vi "test_VISA Close.vi"(8 "error in (no error)":errorcluster, 11 "TestCase in":refnum<class "Instrument Addon Serial Protocols Unit Tests.lvclass">) -> (0 "error out":errorcluster, 3 "TestCase out":refnum<class "Instrument Addon Serial Protocols Unit Tests.lvclass">)   [LabVIEW 2023, in "Instrument Addon Serial Protocols Unit Tests.lvclass"]
uses:
  Instrument Addon Serial Protocols Unit Tests.lvclass
  <vilib>/addons/_JKI Toolkits/VI Tester/TestCase.llb/TestCase.lvclass
  VISA/VISA.lvclass
  Listener/Listener.lvclass
  Listener/ListenerClassControls/Operation.ctl
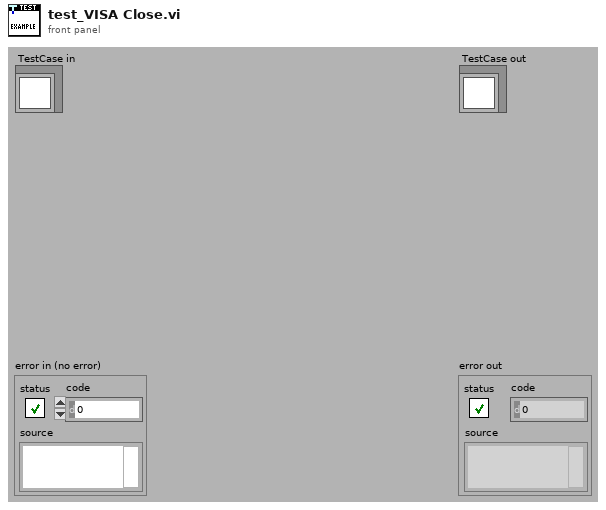
[diagram p1: front panel]
types:
  T1 = typedef "Listener.lvclass/Operation.ctl" = enum16{"Read", "Write"}
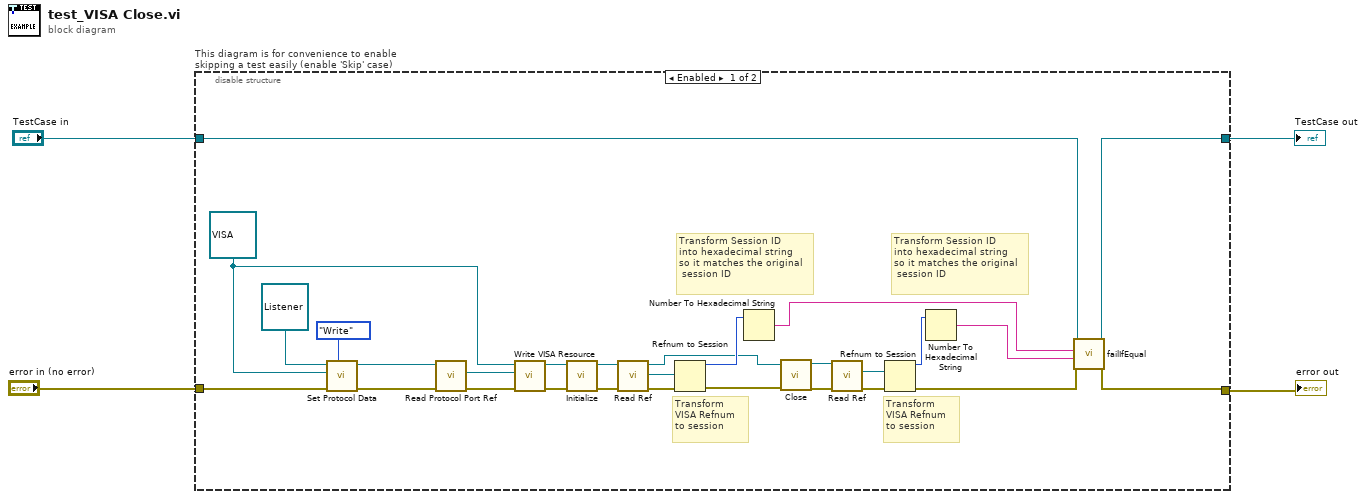
[diagram p0: block diagram]
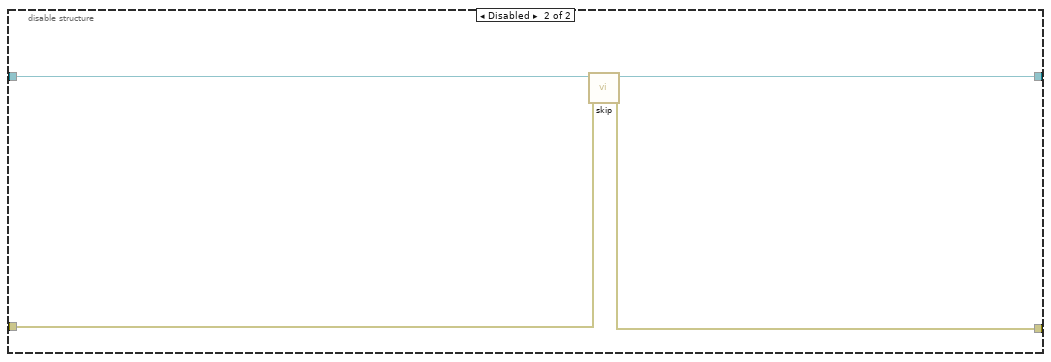
[diagram p2: hidden frame]
diagram:
  n1 = disable-structure "This diagram is for convenience to enable skipping a test easily (enable 'Skip' case)" shown="Enabled" {
    disable-tunnel: "TestCase in" -> [w32 w36]
    disable-tunnel: [w31 w34] -> w1
    disable-tunnel: [w30 w35] -> w3
    disable-tunnel: "error in (no error)" -> [w27 w33]
    frame Enabled {
      w26 = refnum<class "VISA.lvclass"> refnum ("Protocols.lvlib:VISA.lvclass")
      # "Transform Session ID \ninto hexadecimal string\nso it matches the original\n session ID"
      # "Transform \nVISA Refnum \nto session"
      # "Transform Session ID \ninto hexadecimal string\nso it matches the original\n session ID"
      # "Transform \nVISA Refnum \nto session"
      n2 = call "Set Protocol Data.vi"("Operation"=Operation."Write", "error in (no error)"=w27, "Protocols.lvlib:Protocol Parent.lvclass"=w26, "Listener In.lvclass"=refnum<class "Listener.lvclass"> refnum ("Listener.lvclass")) -> ("error out"=w7:errorcluster, "Listener Out.lvclass"=w8:refnum<class "Listener.lvclass">)  [unwired: 6 in]
      n3 = call "Read Protocol Port Ref.vi"("error in (no error)"=w7, "Listener in"=w8) -> ("error out"=w6:errorcluster, "Protocol Port Ref"=w5:refnum<visa-resource-name>)  [unwired: 7 in, 1 out]
      n4 = call "Write VISA Resource.vi"("error in (no error)"=w6, "VISA Resource"=w5, "VISA in"=w26) -> ("error out"=w25:errorcluster, "VISA out"=w24:refnum<class "VISA.lvclass">)  [unwired: 7 in]
      n5 = call-dynamic "Initialize.vi"("error in (no error)"=w25, "VISA in"=w24) -> ("error out"=w23:errorcluster, "VISA out"=w22:refnum<class "VISA.lvclass">)  [unwired: 8 in]
      n6 = call "Read Ref.vi"("error in (no error)"=w23, "VISA in"=w22) -> ("error out"=w18:errorcluster, "Ref"=w21:refnum<visa-resource-name>, "VISA out"=w9:refnum<class "VISA.lvclass">)  [unwired: 7 in]
      n7 = Refnum to Session(4:w18, 7:w21) -> (0:w17:errorcluster, 3:w20:u64)
      n8 = Number To Hexadecimal String(2:w20) -> (0:w10:string)  [unwired: 1 in]
      n9 = call-dynamic "Close.vi"("error in (no error)"=w17, "VISA in"=w9) -> ("error out"=w16:errorcluster, "VISA out"=w19:refnum<class "VISA.lvclass">)  [unwired: 8 in]
      n10 = call "Read Ref.vi"("error in (no error)"=w16, "VISA in"=w19) -> ("error out"=w15:errorcluster, "Ref"=w13:refnum<visa-resource-name>)  [unwired: 7 in, 1 out]
      n11 = Refnum to Session(4:w15, 7:w13) -> (0:w14:errorcluster, 3:w12:u64)
      n12 = Number To Hexadecimal String(2:w12) -> (0:w11:string)  [unwired: 1 in]
      n13 = call-dynamic "failIfEqual.vi"("error in (no error)"=w14, "y"=w11, "x"=w10, "TestCase in"=w32) -> ("error out"=w30:errorcluster, "TestCase out"=w31:refnum<class "Instrument Addon Serial Protocols Unit Tests.lvclass">)  [unwired: 6 in]
    }
    frame Disabled {
      # "skip test result while test is under development"
      n14 = call <vilib>:"skip.vi"("error in (no error)"=w33, "TestCase in"=w36) -> ("error out"=w35:errorcluster, "TestCase out"=w34:refnum<class "Instrument Addon Serial Protocols Unit Tests.lvclass">)  [unwired: 8 in]
    }
  }
  "error out" <- w3
  "TestCase out" <- w1
